vi "ex_prepAOW.vi"(4 "error in (no error)":errorcluster, 5 "Name":string, 7 "Dynamic Data":waveform(dbl)[](array[waveform])) -> (0 "error out":errorcluster, 3 "?":waveform(dbl)[](array[waveform]))   [LabVIEW 2020]
panel:
  in  "?":string="Untitled"
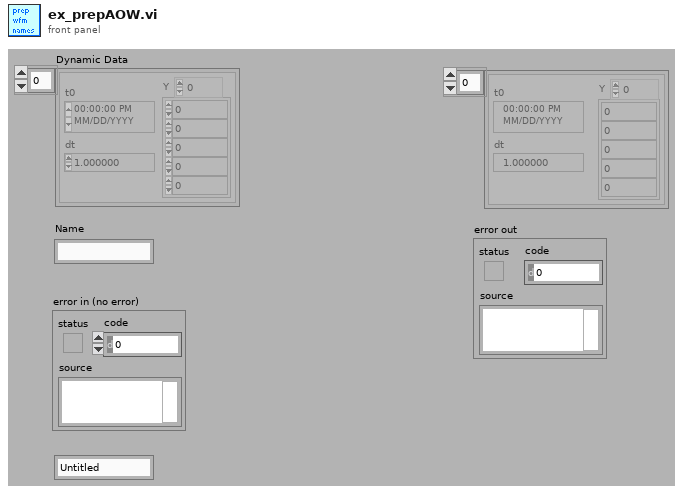
[diagram p1: front panel]
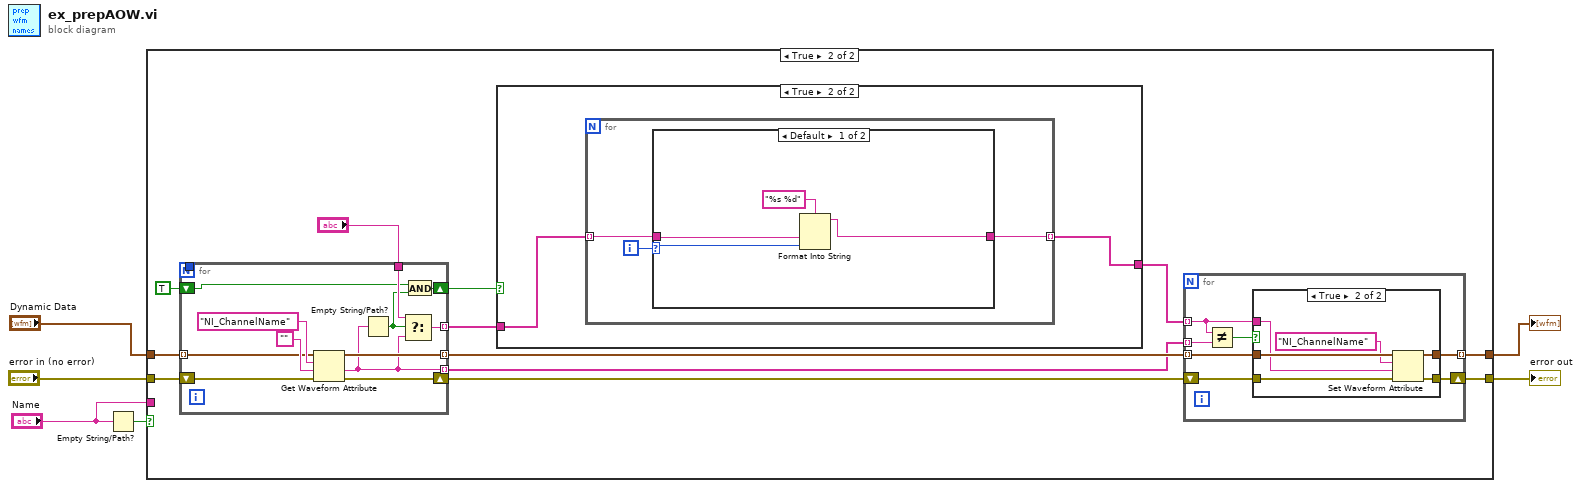
[diagram p0: block diagram]
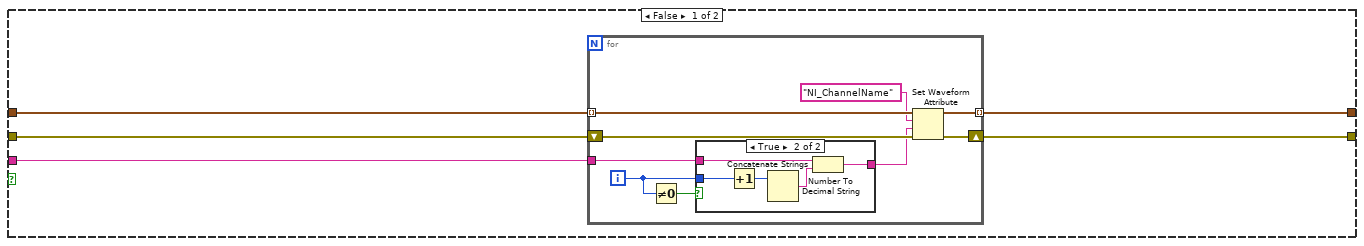
[diagram p2: hidden frame]
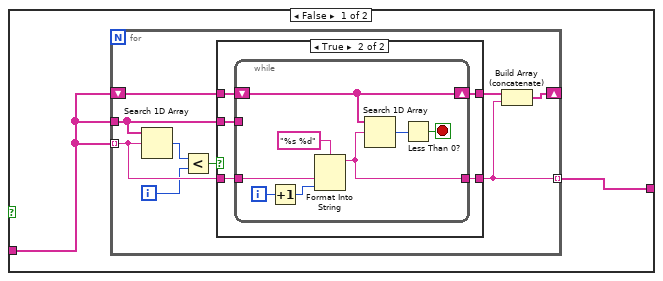
[diagram p4: hidden frame]
diagram:
  n1 = Empty String/Path?(string/path="Name") -> (empty?=w1:bool)
  n2 = case shown="True" w1 {
    tunnel: [w11 w37] -> w6
    tunnel: "error in (no error)" -> [w10 w36]
    tunnel: "Dynamic Data" -> [w9 w34]
    tunnel: [w8 w38] -> w3
    tunnel: "Name" -> [w7 _]
    frame False {
      n3 = for {
        tunnel: w9 -> [w20] mode=indexing
        tunnel: [w18] -> w11 mode=indexing
        shift-right: [w17] -> w8
        shift-left: w10 -> [w19]
        tunnel: w7 -> [w16]
        i -> [w12]
        n4 = Not Equal To 0?(x=w12) -> (x != 0?=w13:bool)
        n5 = case shown="True" w13 {
          tunnel: w16 -> [w21 w26]
          tunnel: w12 -> [_ w25]
          tunnel: [w21 w23] -> w14
          frame False {
          }
          frame True {
            n6 = Increment(x=w25) -> (x+1=w22:i32)
            n7 = Number To Decimal String(number=w22) -> (decimal integer string=w24:string)  [unwired: 1 out]
            n8 = Concatenate Strings(w26, w24) -> (w23:string)
          }
        }
        n9 = Set Waveform Attribute(4:w19, 5:w14, 6:"NI_ChannelName" ("name"), 7:w20) -> (0:w17:errorcluster, 3:w18:waveform(dbl))  [unwired: 1 out]
      }
    }
    frame True {
      n10 = for {
        N -> [w81]
        tunnel: w34 -> [w85] mode=indexing
        tunnel: [w84] -> w33 mode=indexing
        shift-right: [w82] -> w35
        shift-left: w36 -> [w83]
        tunnel: [w79] -> w32 mode=indexing
        tunnel: [w81] -> _
        tunnel: "?" -> [w80]
        tunnel: [w78] -> w30 mode=indexing
        shift-right: [w76] -> w27
        shift-left: TRUE -> [w75]
        n11 = Get Waveform Attribute(4:w83, 5:"", 6:"NI_ChannelName" ("name"), 7:w85) -> (0:w82:errorcluster, 1:w79:string, 3:w84:waveform(dbl))  [unwired: 1 out]
        n12 = Empty String/Path?(string/path=w79) -> (empty?=w77:bool)
        n13 = Select(t=w80, s=w77, f=w79) -> (s? t:f=w78:string)
        n14 = And(x=w75, y=w77) -> (x .and. y?=w76:bool)
      }
      n15 = case shown="True" w27 {
        tunnel: [w40 w65] -> w31
        tunnel: w30 -> [w39 w66]
        frame False {
          n16 = for {
            tunnel: w39 -> [w49]
            tunnel: w39 -> [w48] mode=indexing
            shift-right: [w46] -> _
            shift-left: w39 -> [w47]
            tunnel: [w41] -> w40 mode=indexing
            i -> [w44]
            n17 = Search 1D Array(1D array=w49, element=w48) -> (index of element=w43:i32)  [unwired: 1 out]
            n18 = Less?(x=w43, y=w44) -> (x < y?=w42:bool)
            n19 = case shown="True" w42 {
              tunnel: w49 -> [_ w56]
              tunnel: w48 -> [w51 w55]
              tunnel: [w51 w54] -> w41
              tunnel: w47 -> [w50 w53]
              tunnel: [w50 w52] -> w45
              frame False {
              }
              frame True {
                n20 = while {
                  tunnel: w56 -> [_]
                  tunnel: w55 -> [w63]
                  tunnel: [w60] -> w54
                  shift-right: [w57] -> w52
                  shift-left: w53 -> [w57]
                  i -> [w59]
                  stop <- w61 stop-if-true
                  n21 = Increment(x=w59) -> (x+1=w58:i32)
                  n22 = Format Into String(format string="%s %d", w63, w58) -> (resulting string=w60:string)  [unwired: 2 in, 1 out]
                  n23 = Search 1D Array(1D array=w57, element=w60) -> (index of element=w62:i32)  [unwired: 1 out]
                  n24 = Less Than 0?(x=w62) -> (x < 0?=w61:bool)
                }
              }
            }
            n25 = Build Array (concatenate)(w45, w41) -> (w46:string[])
          }
        }
        frame True {
          n26 = for {
            tunnel: w66 -> [w68] mode=indexing
            tunnel: [w67] -> w65 mode=indexing
            i -> [w69]
            n27 = case shown="Default" w69 {
              selector: w69 -> [w70 _]
              tunnel: w68 -> [w72 w74]
              tunnel: [w71 w74] -> w67
              frame Default {
                n28 = Format Into String(format string="%s %d", w72, w70) -> (resulting string=w71:string)  [unwired: 2 in, 1 out]
              }
              frame 0 {
              }
            }
          }
        }
      }
      n29 = for {
        tunnel: w33 -> [w91] mode=indexing
        tunnel: [w94] -> w37 mode=indexing
        shift-right: [w93] -> w38
        shift-left: w35 -> [w92]
        tunnel: w31 -> [w90] mode=indexing
        tunnel: w32 -> [w89] mode=indexing
        n30 = Not Equal?(x=w90, y=w89) -> (x != y?=w88:bool)
        n31 = case shown="True" w88 {
          tunnel: [w96 w102] -> w94
          tunnel: [w95 w101] -> w93
          tunnel: w92 -> [w95 w100]
          tunnel: w91 -> [w96 w99]
          tunnel: w90 -> [_ w97]
          frame False {
          }
          frame True {
            n32 = Set Waveform Attribute(4:w100, 5:w97, 6:"NI_ChannelName" ("name"), 7:w99) -> (0:w101:errorcluster, 3:w102:waveform(dbl))  [unwired: 1 out]
          }
        }
      }
    }
  }
  "?" <- w6
  "error out" <- w3
